vi "Read Read Only.vi"(8 "error in (no error)":errorcluster, 11 "Const_I16 in":refnum<class "Const_I16.lvclass">) -> (0 "error out":errorcluster, 2 "Read Only":bool, 3 "Const_I16 out":refnum<class "Const_I16.lvclass">)   [LabVIEW 2021, in "Const_I16.lvclass"]
uses:
  Const_I16.lvclass
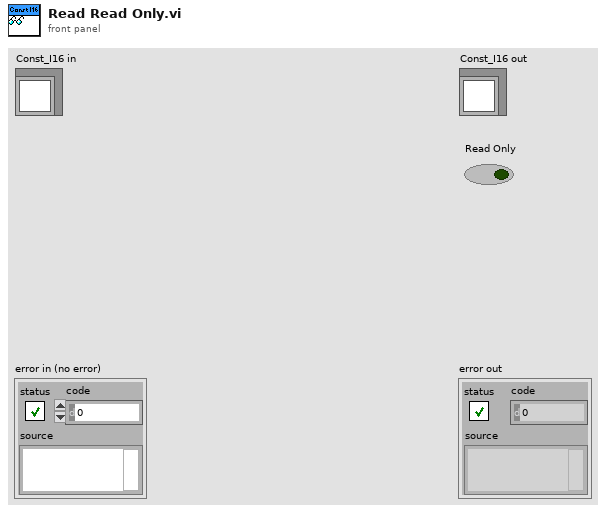
[diagram p1: front panel]
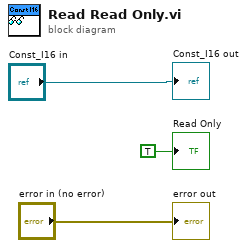
[diagram p0: block diagram]
diagram:
  "error out" <- "error in (no error)"
  "Const_I16 out" <- "Const_I16 in"
  "Read Only" <- TRUE ("Read Only")
